vi "get angle index.vi"(6 "Center Post Pulse":cluster{"X":dbl, "Y":dbl}={"X"=72700.0, "Y"=72100.0}, 7 "Vert_Dist":cluster{"X":dbl, "Y":dbl}={"X"=245000.0, "Y"=245000.0}, 10 "y angle":dbl[](array[numeric]), 11 "x angle":dbl[](array[numeric])) -> (0 "y dist":dbl[](array[numeric]), 1 "x  dist":dbl[](array[numeric]), 2 "angle":dbl[](array[numeric]), 3 "appended array":dbl[][](array[numeric]), 4 "y":i32[][](array[numeric]), 5 "x":i32[][](array[numeric]))   [LabVIEW 2015]
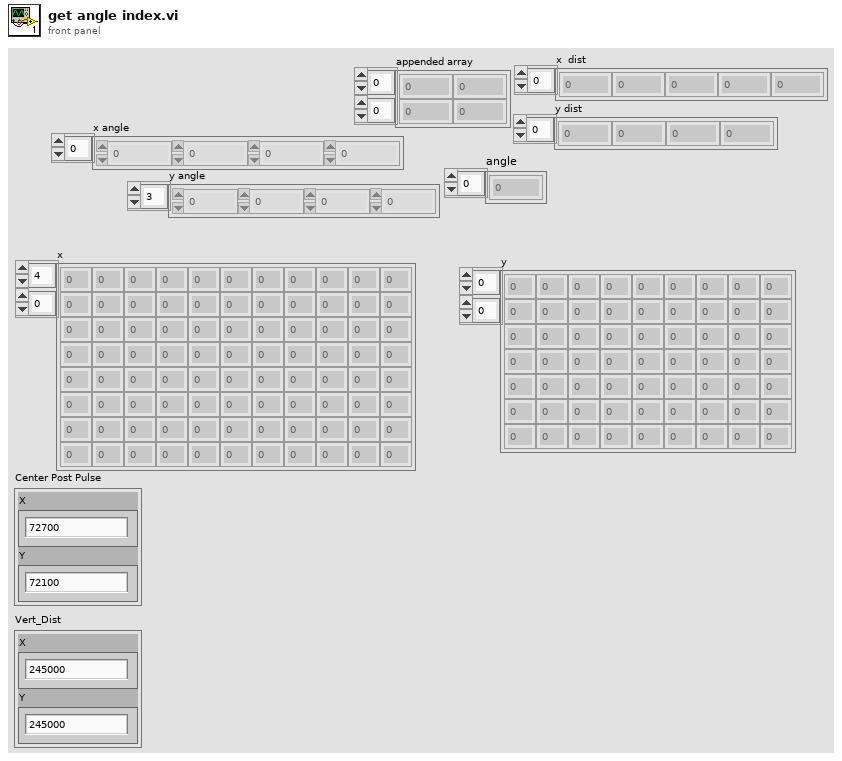
[diagram p1: front panel]
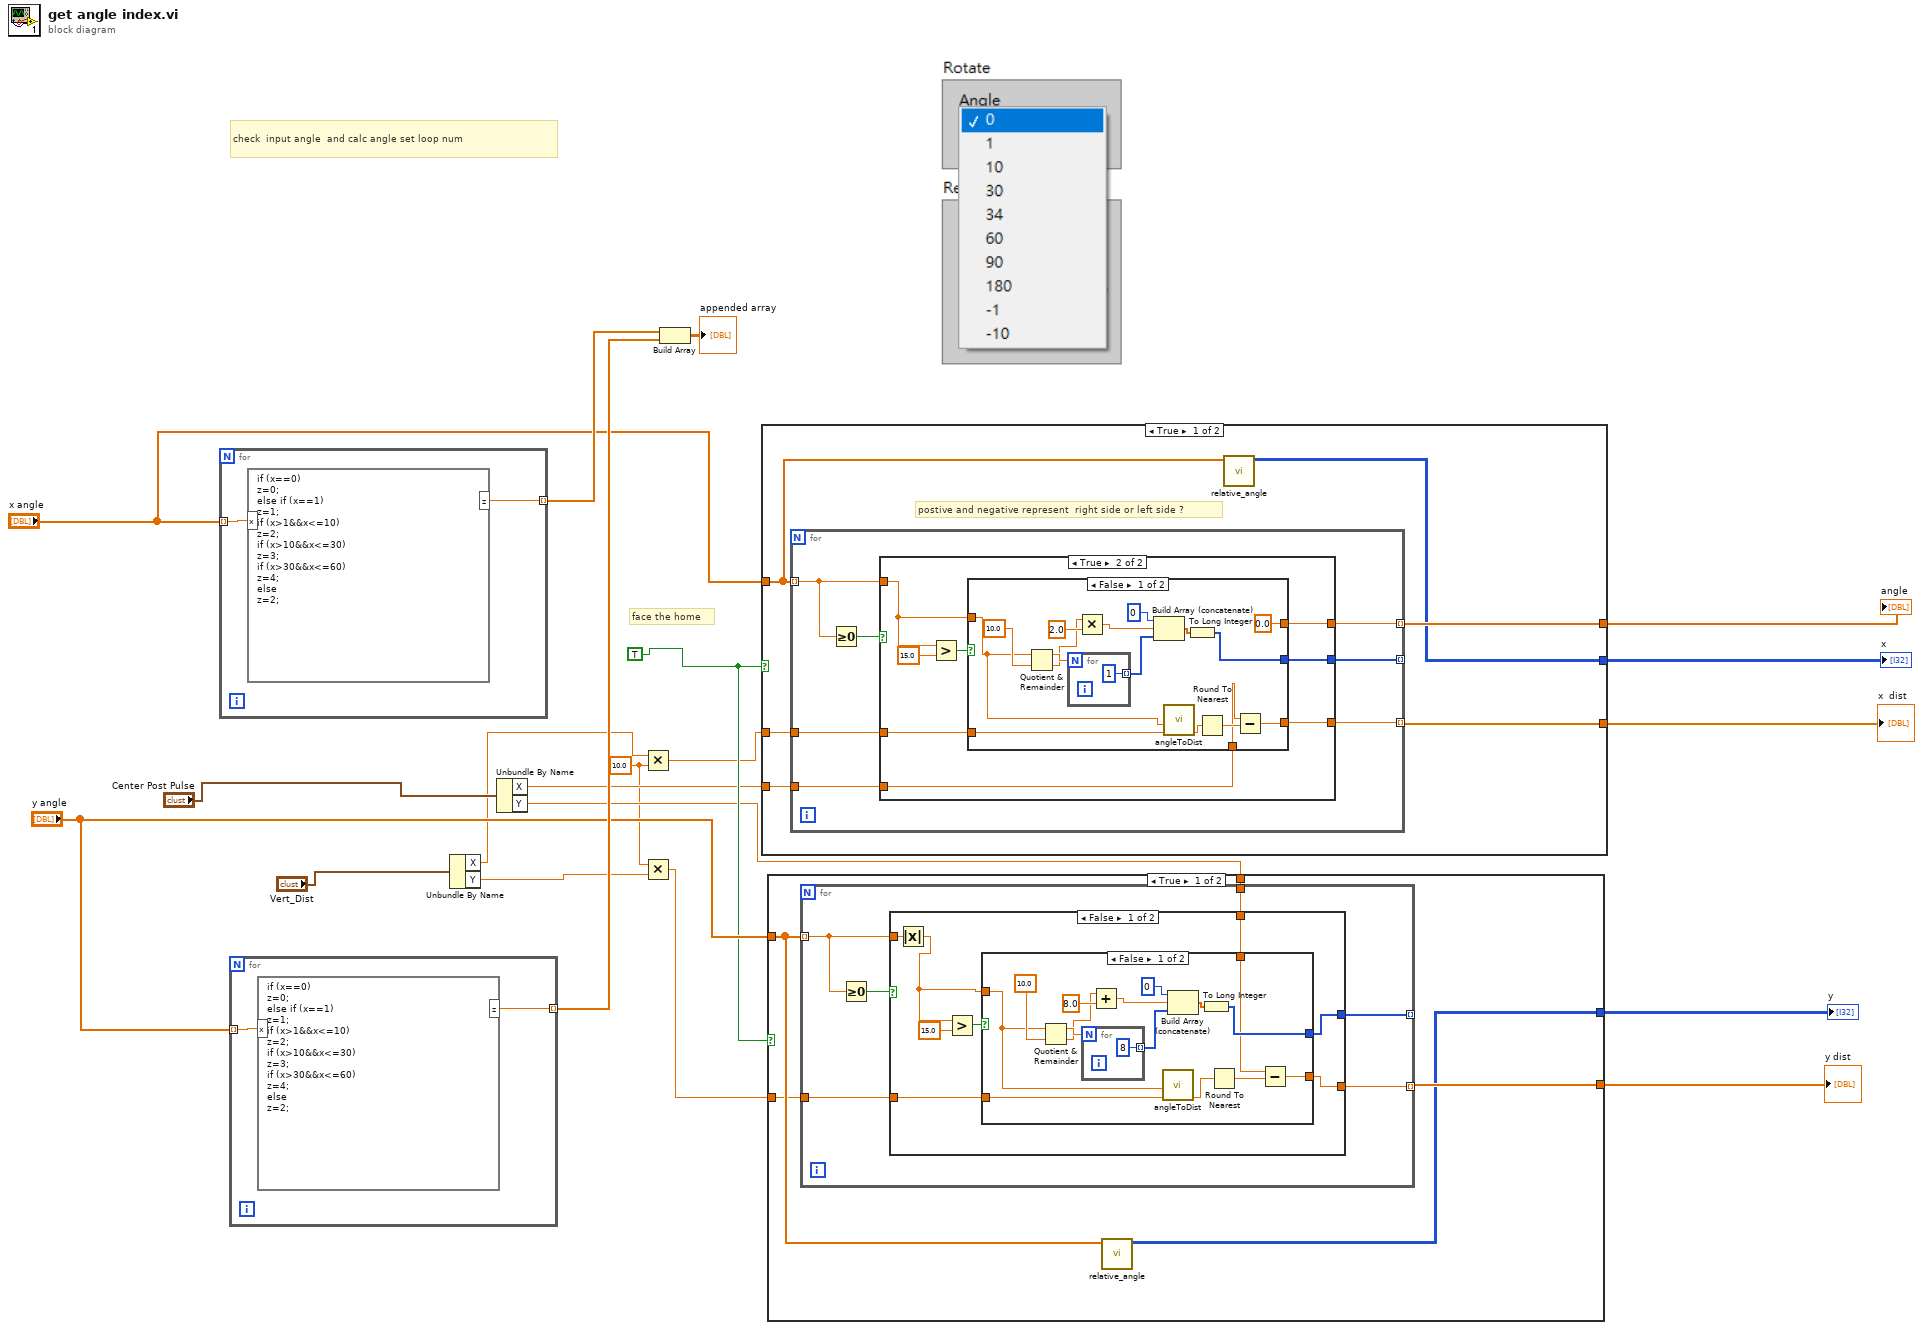
[diagram p0: block diagram]
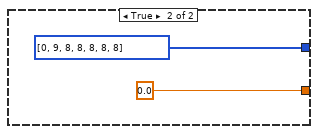
[diagram p2: hidden frame]
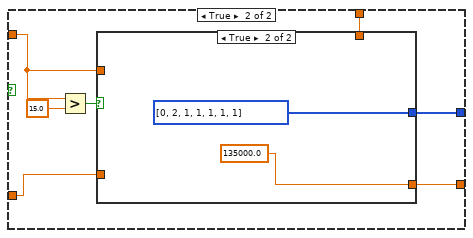
[diagram p3: hidden frame]
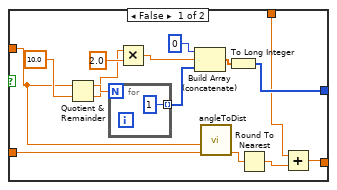
[diagram p4: hidden frame]
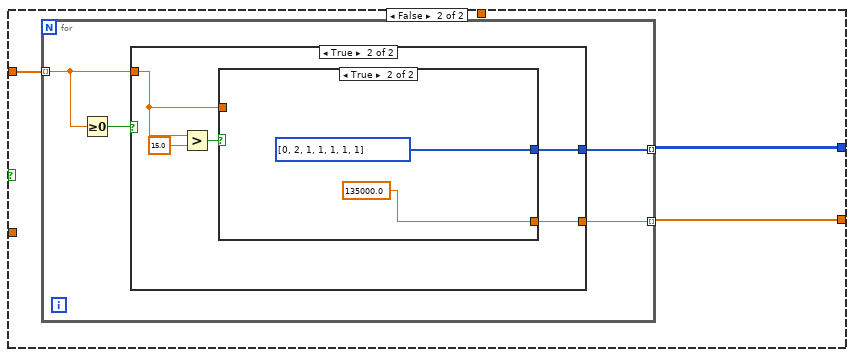
[diagram p5: hidden frame]
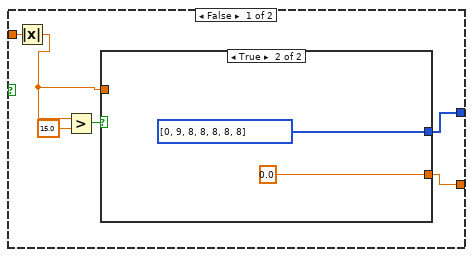
[diagram p6: hidden frame]
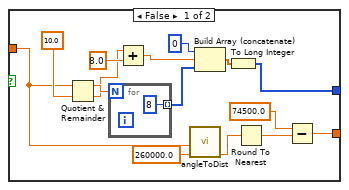
[diagram p7: hidden frame]
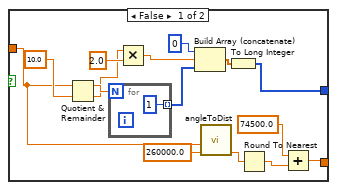
[diagram p8: hidden frame]
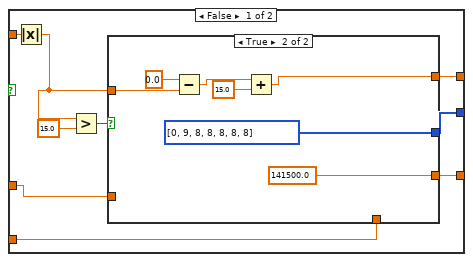
[diagram p9: hidden frame]
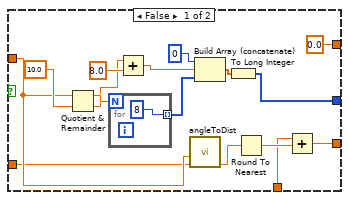
[diagram p10: hidden frame]
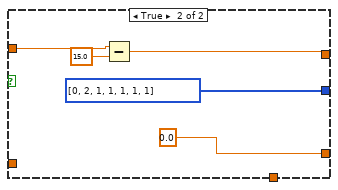
[diagram p11: hidden frame]
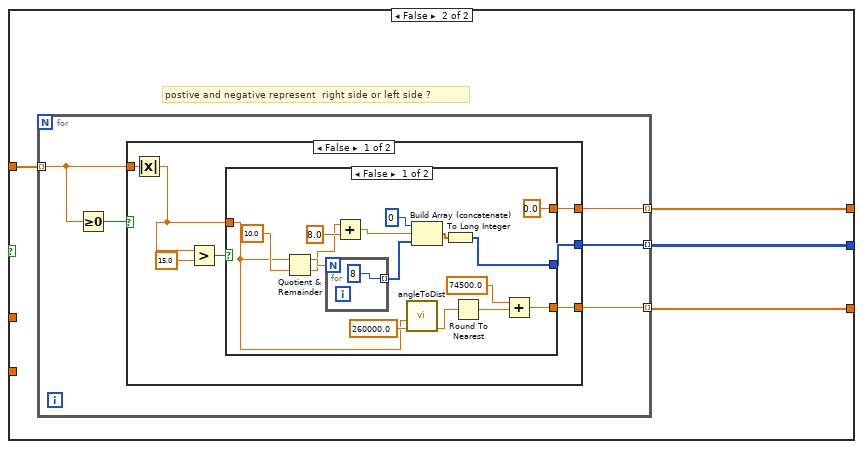
[diagram p12: hidden frame]
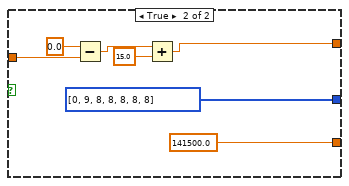
[diagram p13: hidden frame]
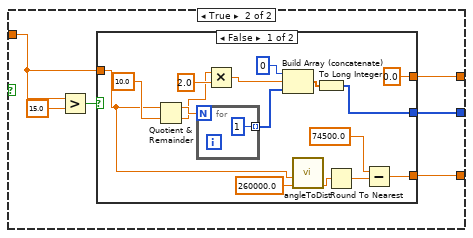
[diagram p14: hidden frame]
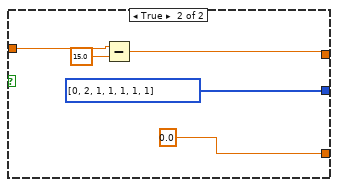
[diagram p15: hidden frame]
diagram:
  w1 = 10.0 ("y")
  w10 = TRUE
  # "face the home"
  # "check  input angle  and calc angle set loop num"
  n1 = for {
    tunnel: "x angle" -> [w22] mode=indexing
    tunnel: [w21] -> w20 mode=indexing
    n2 = formula code="if (x==0)\nz=0;\nelse if (x==1)\nz=1;\nif (x>1&&x<=10)\nz=2;\nif (x>10&&x<=30)\nz=3;\nif (x>30&&x<=60)\nz=4;\nelse\nz=2;"("x"=w22) -> ("z"=w21:dbl)
  }
  n3 = for {
    tunnel: [w24] -> w19 mode=indexing
    tunnel: "y angle" -> [w23] mode=indexing
    n4 = formula code="if (x==0)\nz=0;\nelse if (x==1)\nz=1;\nif (x>1&&x<=10)\nz=2;\nif (x>10&&x<=30)\nz=3;\nif (x>30&&x<=60)\nz=4;\nelse\nz=2;"("x"=w23) -> ("z"=w24:dbl)
  }
  n5 = Unbundle By Name("Vert_Dist") -> ("X"=w5:dbl, "Y"=w3:dbl)
  n6 = Unbundle By Name("Center Post Pulse") -> ("X"=w8:dbl, "Y"=w7:dbl)
  n7 = Multiply(x=w5, y=w1) -> (x*y=w4:dbl)
  n8 = Multiply(x=w1, y=w3) -> (x*y=w2:dbl)
  n9 = Build Array(w20, w19) -> (→"appended array":dbl[][])
  n10 = case shown="True" w10 {
    tunnel: "x angle" -> [w28 w104]
    tunnel: [w27 w103] -> w15
    tunnel: [w30 w102] -> w13
    tunnel: [w29 w101] -> w11
    tunnel: w8 -> [w26 _]
    tunnel: w4 -> [w25 _]
    frame True {
      # "postive and negative represent  right side or left side ?"
      n11 = for {
        tunnel: w28 -> [w36] mode=indexing
        tunnel: [w35] -> _ mode=indexing
        tunnel: [w34] -> w30 mode=indexing
        tunnel: [w33] -> w29 mode=indexing
        tunnel: w26 -> [w32]
        tunnel: w25 -> [w31]
        n12 = Greater Or Equal To 0?(x=w36) -> (x >= 0?=w37:bool)
        n13 = case shown="True" w37 {
          tunnel: w36 -> [w42 w76]
          tunnel: [w44 w75] -> w35
          tunnel: [w43 w74] -> w34
          tunnel: [w40 w73] -> w33
          tunnel: w32 -> [w39 w72]
          tunnel: w31 -> [w38 w71]
          frame False {
            n14 = Absolute Value(x=w42) -> (abs(x)=w41:dbl)
            n15 = Greater?(x=w41, y=15.0) -> (0:w45:bool)
            n16 = case shown="True" w45 {
              tunnel: [w59 i32[] [0, 9, 8, 8, 8, 8, 8]] -> w44
              tunnel: w41 -> [w53 w68]
              tunnel: [w51 141500.0] -> w43
              tunnel: [0.0 w64] -> w40
              tunnel: w39 -> [w48 _]
              tunnel: w38 -> [w47 _]
              frame False {
                n17 = Quotient & Remainder(x=w53, y=10.0) -> (x-y*floor(x/y)=w62:dbl, floor(x/y)=w54:dbl)
                n18 = for {
                  N: w62 -> [_]
                  tunnel: [8] -> w61 mode=indexing
                }
                n19 = Add(x=w54, y=8.0) -> (x+y=w56:dbl)
                n20 = call "angleToDist.vi"("y"=w47, "angle"=w53) -> ("tan(x)"=w52:dbl)  [unwired: 8 in, 1 out]
                n21 = Build Array (concatenate)(0, w56, w61) -> (w60:dbl[])
                n22 = To Long Integer(number=w60) -> (32bit integer=w59:i32[])
                n23 = Round To Nearest(number=w52) -> (nearest integer value=w50:dbl)
                n24 = Add(x=w48, y=w50) -> (x+y=w51:dbl)
              }
              frame True {
                n25 = Subtract(x=0.0, y=w68) -> (x-y=w66:dbl)
                n26 = Add(x=w66, y=15.0) -> (x+y=w64:dbl)
              }
            }
          }
          frame True {
            n27 = Greater?(x=w76, y=15.0) -> (0:w77:bool)
            n28 = case shown="False" w77 {
              tunnel: [w91 i32[] [0, 2, 1, 1, 1, 1, 1]] -> w75
              tunnel: w76 -> [w85 w98]
              tunnel: [w83 0.0] -> w74
              tunnel: [0.0 w96] -> w73
              tunnel: w72 -> [w80 _]
              tunnel: w71 -> [w79 _]
              frame False {
                n29 = Quotient & Remainder(x=w85, y=10.0) -> (x-y*floor(x/y)=w94:dbl, floor(x/y)=w86:dbl)
                n30 = for {
                  N: w94 -> [_]
                  tunnel: [1] -> w93 mode=indexing
                }
                n31 = Multiply(x=w86, y=2.0) -> (x*y=w88:dbl)
                n32 = Build Array (concatenate)(0, w88, w93) -> (w92:dbl[])
                n33 = call "angleToDist.vi"("y"=w79, "angle"=w85) -> ("tan(x)"=w84:dbl)  [unwired: 8 in, 1 out]
                n34 = To Long Integer(number=w92) -> (32bit integer=w91:i32[])
                n35 = Round To Nearest(number=w84) -> (nearest integer value=w82:dbl)
                n36 = Subtract(x=w80, y=w82) -> (x-y=w83:dbl)
              }
              frame True {
                n37 = Subtract(x=w98, y=15.0) -> (x-y=w96:dbl)
              }
            }
          }
        }
      }
      n38 = call "relative_angle.vi"("y angle"=w28) -> ("Array"=w27:i32[][])  [unwired: 10 in]
    }
    frame False {
      # "postive and negative represent  right side or left side ?"
      n39 = for {
        tunnel: w104 -> [w108] mode=indexing
        tunnel: [w107] -> w103 mode=indexing
        tunnel: [w106] -> w102 mode=indexing
        tunnel: [w105] -> w101 mode=indexing
        n40 = Greater Or Equal To 0?(x=w108) -> (x >= 0?=w109:bool)
        n41 = case shown="False" w109 {
          tunnel: w108 -> [w112 w144]
          tunnel: [w114 w143] -> w107
          tunnel: [w113 w142] -> w106
          tunnel: [w110 w141] -> w105
          frame False {
            n42 = Absolute Value(x=w112) -> (abs(x)=w111:dbl)
            n43 = Greater?(x=w111, y=15.0) -> (0:w115:bool)
            n44 = case shown="False" w115 {
              tunnel: [w129 i32[] [0, 9, 8, 8, 8, 8, 8]] -> w114
              tunnel: w111 -> [w122 w138]
              tunnel: [w120 141500.0] -> w113
              tunnel: [0.0 w134] -> w110
              frame False {
                n45 = Quotient & Remainder(x=w122, y=10.0) -> (x-y*floor(x/y)=w132:dbl, floor(x/y)=w124:dbl)
                n46 = for {
                  N: w132 -> [_]
                  tunnel: [8] -> w131 mode=indexing
                }
                n47 = Add(x=w124, y=8.0) -> (x+y=w126:dbl)
                n48 = call "angleToDist.vi"("y"=260000.0, "angle"=w122) -> ("tan(x)"=w121:dbl)  [unwired: 8 in, 1 out]
                n49 = Build Array (concatenate)(0, w126, w131) -> (w130:dbl[])
                n50 = To Long Integer(number=w130) -> (32bit integer=w129:i32[])
                n51 = Round To Nearest(number=w121) -> (nearest integer value=w118:dbl)
                n52 = Add(x=74500.0, y=w118) -> (x+y=w120:dbl)
              }
              frame True {
                n53 = Subtract(x=0.0, y=w138) -> (x-y=w136:dbl)
                n54 = Add(x=w136, y=15.0) -> (x+y=w134:dbl)
              }
            }
          }
          frame True {
            n55 = Greater?(x=w144, y=15.0) -> (0:w145:bool)
            n56 = case shown="False" w145 {
              tunnel: [w159 i32[] [0, 2, 1, 1, 1, 1, 1]] -> w143
              tunnel: w144 -> [w152 w166]
              tunnel: [w150 0.0] -> w142
              tunnel: [0.0 w164] -> w141
              frame False {
                n57 = Quotient & Remainder(x=w152, y=10.0) -> (x-y*floor(x/y)=w162:dbl, floor(x/y)=w154:dbl)
                n58 = for {
                  N: w162 -> [_]
                  tunnel: [1] -> w161 mode=indexing
                }
                n59 = Multiply(x=w154, y=2.0) -> (x*y=w156:dbl)
                n60 = Build Array (concatenate)(0, w156, w161) -> (w160:dbl[])
                n61 = call "angleToDist.vi"("y"=260000.0, "angle"=w152) -> ("tan(x)"=w151:dbl)  [unwired: 8 in, 1 out]
                n62 = To Long Integer(number=w160) -> (32bit integer=w159:i32[])
                n63 = Round To Nearest(number=w151) -> (nearest integer value=w148:dbl)
                n64 = Subtract(x=74500.0, y=w148) -> (x-y=w150:dbl)
              }
              frame True {
                n65 = Subtract(x=w166, y=15.0) -> (x-y=w164:dbl)
              }
            }
          }
        }
      }
    }
  }
  "x" <- w15
  "x  dist" <- w13
  "angle" <- w11
  n66 = case shown="True" w10 {
    tunnel: "y angle" -> [w172 w233]
    tunnel: [w171 w232] -> w14
    tunnel: [w173 w231] -> w12
    tunnel: w7 -> [w170 _]
    tunnel: w2 -> [w169 _]
    frame True {
      n67 = for {
        tunnel: w172 -> [w178] mode=indexing
        tunnel: [w177] -> _ mode=indexing
        tunnel: [w176] -> w173 mode=indexing
        tunnel: w170 -> [w175]
        tunnel: w169 -> [w174]
        n68 = Greater Or Equal To 0?(x=w178) -> (x >= 0?=w179:bool)
        n69 = case shown="False" w179 {
          tunnel: w178 -> [w186 w210]
          tunnel: [w182 w209] -> w177
          tunnel: [w183 w208] -> w176
          tunnel: w175 -> [w181 w207]
          tunnel: w174 -> [w180 w206]
          frame False {
            n70 = Absolute Value(x=w186) -> (abs(x)=w185:dbl)
            n71 = Greater?(x=w185, y=15.0) -> (0:w184:bool)
            n72 = case shown="False" w184 {
              tunnel: [w199 i32[] [0, 9, 8, 8, 8, 8, 8]] -> w182
              tunnel: w185 -> [w193 _]
              tunnel: [w191 0.0] -> w183
              tunnel: w181 -> [w189 _]
              tunnel: w180 -> [w188 _]
              frame False {
                n73 = Quotient & Remainder(x=w193, y=10.0) -> (x-y*floor(x/y)=w202:dbl, floor(x/y)=w194:dbl)
                n74 = for {
                  N: w202 -> [_]
                  tunnel: [8] -> w201 mode=indexing
                }
                n75 = Add(x=w194, y=8.0) -> (x+y=w196:dbl)
                n76 = call "angleToDist.vi"("y"=w188, "angle"=w193) -> ("tan(x)"=w192:dbl)  [unwired: 8 in, 1 out]
                n77 = Build Array (concatenate)(0, w196, w201) -> (w200:dbl[])
                n78 = To Long Integer(number=w200) -> (32bit integer=w199:i32[])
                n79 = Round To Nearest(number=w192) -> (nearest integer value=w190:dbl)
                n80 = Subtract(x=w189, y=w190) -> (x-y=w191:dbl)
              }
              frame True {
              }
            }
          }
          frame True {
            n81 = Greater?(x=w210, y=15.0) -> (0:w211:bool)
            n82 = case shown="True" w211 {
              tunnel: [w217 i32[] [0, 2, 1, 1, 1, 1, 1]] -> w209
              tunnel: w210 -> [w219 _]
              tunnel: [w216 135000.0] -> w208
              tunnel: w207 -> [w214 _]
              tunnel: w206 -> [w213 _]
              frame False {
                n83 = Quotient & Remainder(x=w219, y=10.0) -> (x-y*floor(x/y)=w227:dbl, floor(x/y)=w220:dbl)
                n84 = for {
                  N: w227 -> [_]
                  tunnel: [1] -> w226 mode=indexing
                }
                n85 = Multiply(x=w220, y=2.0) -> (x*y=w222:dbl)
                n86 = Build Array (concatenate)(0, w222, w226) -> (w225:dbl[])
                n87 = call "angleToDist.vi"("y"=w213, "angle"=w219) -> ("tan(x)"=w218:dbl)  [unwired: 8 in, 1 out]
                n88 = To Long Integer(number=w225) -> (32bit integer=w217:i32[])
                n89 = Round To Nearest(number=w218) -> (nearest integer value=w215:dbl)
                n90 = Add(x=w214, y=w215) -> (x+y=w216:dbl)
              }
              frame True {
              }
            }
          }
        }
      }
      n91 = call "relative_angle.vi"("y angle"=w172) -> ("Array"=w171:i32[][])  [unwired: 10 in]
    }
    frame False {
      n92 = for {
        tunnel: w233 -> [w236] mode=indexing
        tunnel: [w235] -> w232 mode=indexing
        tunnel: [w234] -> w231 mode=indexing
        n93 = Greater Or Equal To 0?(x=w236) -> (x >= 0?=w237:bool)
        n94 = case shown="True" w237 {
          tunnel: w236 -> [w242 w264]
          tunnel: [w238 w263] -> w235
          tunnel: [w239 w262] -> w234
          frame False {
            n95 = Absolute Value(x=w242) -> (abs(x)=w241:dbl)
            n96 = Greater?(x=w241, y=15.0) -> (0:w240:bool)
            n97 = case shown="True" w240 {
              tunnel: [w255 i32[] [0, 9, 8, 8, 8, 8, 8]] -> w238
              tunnel: w241 -> [w248 _]
              tunnel: [w246 0.0] -> w239
              frame False {
                n98 = Quotient & Remainder(x=w248, y=10.0) -> (x-y*floor(x/y)=w258:dbl, floor(x/y)=w250:dbl)
                n99 = for {
                  N: w258 -> [_]
                  tunnel: [8] -> w257 mode=indexing
                }
                n100 = Add(x=w250, y=8.0) -> (x+y=w252:dbl)
                n101 = call "angleToDist.vi"("y"=260000.0, "angle"=w248) -> ("tan(x)"=w247:dbl)  [unwired: 8 in, 1 out]
                n102 = Build Array (concatenate)(0, w252, w257) -> (w256:dbl[])
                n103 = To Long Integer(number=w256) -> (32bit integer=w255:i32[])
                n104 = Round To Nearest(number=w247) -> (nearest integer value=w244:dbl)
                n105 = Subtract(x=74500.0, y=w244) -> (x-y=w246:dbl)
              }
              frame True {
              }
            }
          }
          frame True {
            n106 = Greater?(x=w264, y=15.0) -> (0:w265:bool)
            n107 = case shown="True" w265 {
              tunnel: [w270 i32[] [0, 2, 1, 1, 1, 1, 1]] -> w263
              tunnel: w264 -> [w273 _]
              tunnel: [w269 135000.0] -> w262
              frame False {
                n108 = Quotient & Remainder(x=w273, y=10.0) -> (x-y*floor(x/y)=w281:dbl, floor(x/y)=w274:dbl)
                n109 = for {
                  N: w281 -> [_]
                  tunnel: [1] -> w280 mode=indexing
                }
                n110 = Multiply(x=w274, y=2.0) -> (x*y=w276:dbl)
                n111 = Build Array (concatenate)(0, w276, w280) -> (w279:dbl[])
                n112 = call "angleToDist.vi"("y"=260000.0, "angle"=w273) -> ("tan(x)"=w271:dbl)  [unwired: 8 in, 1 out]
                n113 = To Long Integer(number=w279) -> (32bit integer=w270:i32[])
                n114 = Round To Nearest(number=w271) -> (nearest integer value=w268:dbl)
                n115 = Add(x=74500.0, y=w268) -> (x+y=w269:dbl)
              }
              frame True {
              }
            }
          }
        }
      }
    }
  }
  "y" <- w14
  "y dist" <- w12
